vi "main.vi"() -> ()   [LabVIEW 2012]
uses:
  <vilib>/SAPHIR/ViBox - XControls/XTab/XTab.xctl
  <vilib>/GPower/VIRegister/Library/Typedefs/RegisterType.ctl
  <vilib>/GPower/VIRegister/Library/QManager/CreateRegister.vi
  <vilib>/GPower/VIRegister/Library/SubVIs/FindRegisterData.vi
  <vilib>/GPower/VIRegister/Library/SubVIs/WriteSub.vi
  <vilib>/GPower/VIRegister/Library/QManager/ReleaseRegister.vi
  <vilib>/GPower/Error/Library/IsError.vi
  <vilib>/GPower/VIRegister/Library/QManager/ReleaseAll.vi
  <vilib>/GPower/VIRegister/Library/QManager/QManagerAction.vi
  <vilib>/GPower/VIRegister/Library/QManager/GetRegisterData.vi
  <vilib>/GPower/Error/Library/SetError.vi
  <vilib>/GPower/Error/Library/FilterCodes.vi
  <vilib>/GPower/Error/Library/Filter/FilterMulti.vi
  <vilib>/GPower/Error/Library/ErrorType.vi
  <vilib>/GPower/Error/Library/SplitAppended.vi
  <vilib>/GPower/Error/Library/SubVIs/ExplanationToError.vi
  src/top/gloable.vi
  <vilib>/GPower/VIRegister/Library/QManager/GetQName.vi
  <vilib>/GPower/VIRegister/Library/QManager/StartQManager.vi
  <vilib>/Utility/config.llb/Read Key (String).vi
  <vilib>/Utility/config.llb/Read Key (U32).vi
  <vilib>/Utility/error.llb/Trim Whitespace.vi
  <vilib>/dlg_ctls.llb/Space Constant.vi
  <vilib>/Utility/error.llb/Error Code Database.vi
  <vilib>/GPower/Error/Library/SubVIs/SetStatus.vi
  <vilib>/GPower/Error/Library/AppendErrors.vi
  <vilib>/GPower/Error/Library/Append/AppendSingle.vi
  <vilib>/GPower/VIRegister/VIRegister.lvlib
  <vilib>/Utility/config.llb/NI_LVConfig.lvlib
panel:
  in  "XTab":refnum<vi>(xcontrol)
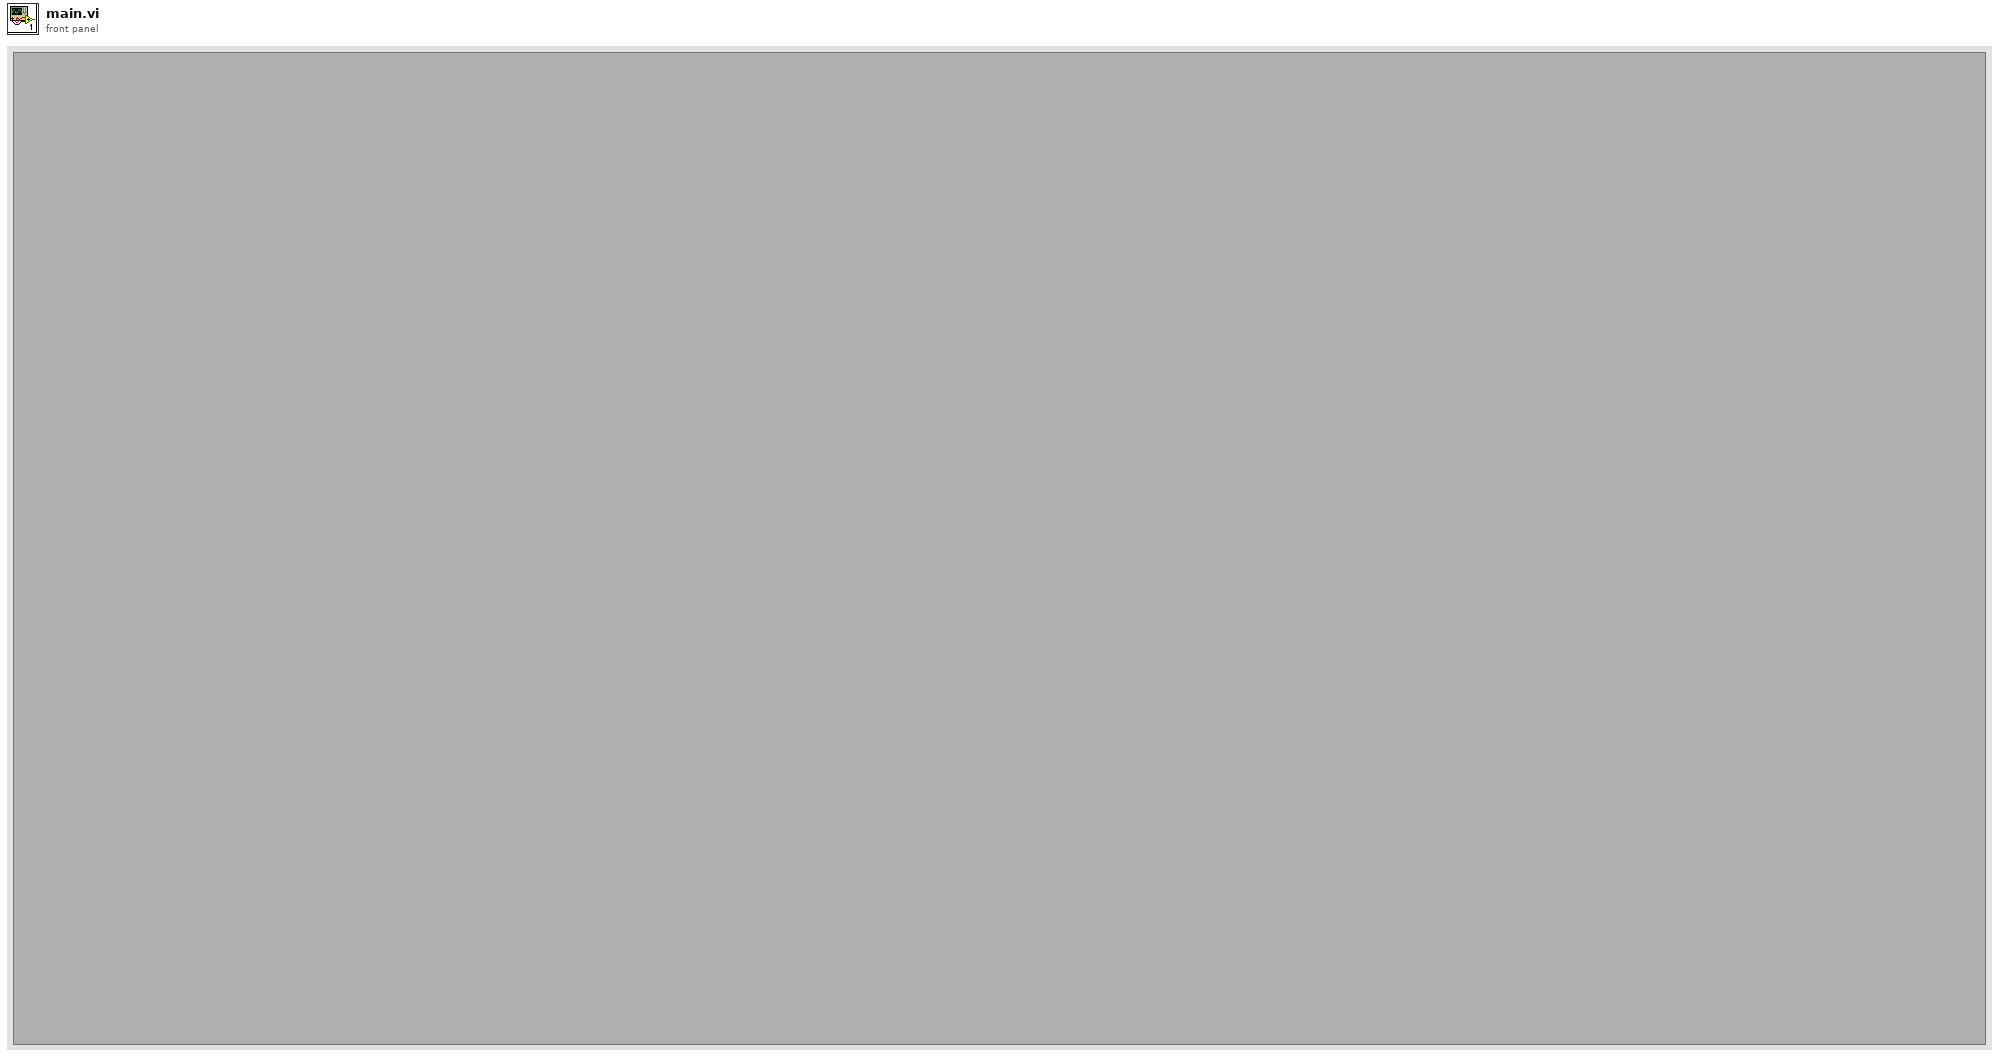
[diagram p1: front panel]
types:
  T1 = enum32{"invalid app kind", "Development System", "Run Time System", "Student Edition", "Embedded LabVIEW", "Evaluation", "Custom"}
  T2 = cluster{" 数据帧名称":string, " 数据":string, "备用操作符":bool, "起始地址":i32, "读写标志":i32, "长度":i32}
  T3 = enum32{"Invalid", "Standard", "Closed", "Hidden", "Minimized", "Maximized"}
  T4 = cluster{"Core":cluster{"Current VI Reference":refnum<vi>, "Close Panel on Exit?":bool}, "事件注册引用句柄":refnum<event-registration>, "XTab":refnum<vi>, "线程数组":refnum<vi>[], "通讯线程":refnum<vi>, "notifier out":refnum<notifier>, "sample_page":refnum<vi>, "queue out":refnum<queue>, "板卡":u32[], "txt引用":refnum<vi>}
  T5 = cluster{"Core":cluster{"Current VI Reference":refnum<vi>, "Close Panel on Exit?":bool}, "事件注册引用句柄":refnum<event-registration>, "XTab":refnum<vi>, "main_page":refnum<vi>, "earth_catch":refnum<vi>, "notifier out":refnum<notifier>, "sample_page":refnum<vi>}
  T6 = cluster{"Current VI Reference":refnum<vi>, "Close Panel on Exit?":bool}
  T7 = typedef "VIRegister.lvlib/RegisterType.ctl" = enum16{"Circular buffer", "FIFO buffer", "LIFO buffer", "Register"}
  T8 = typedef "NI_LVConfig.lvlib/Config Data RefNum.ctl" = refnum<k1>
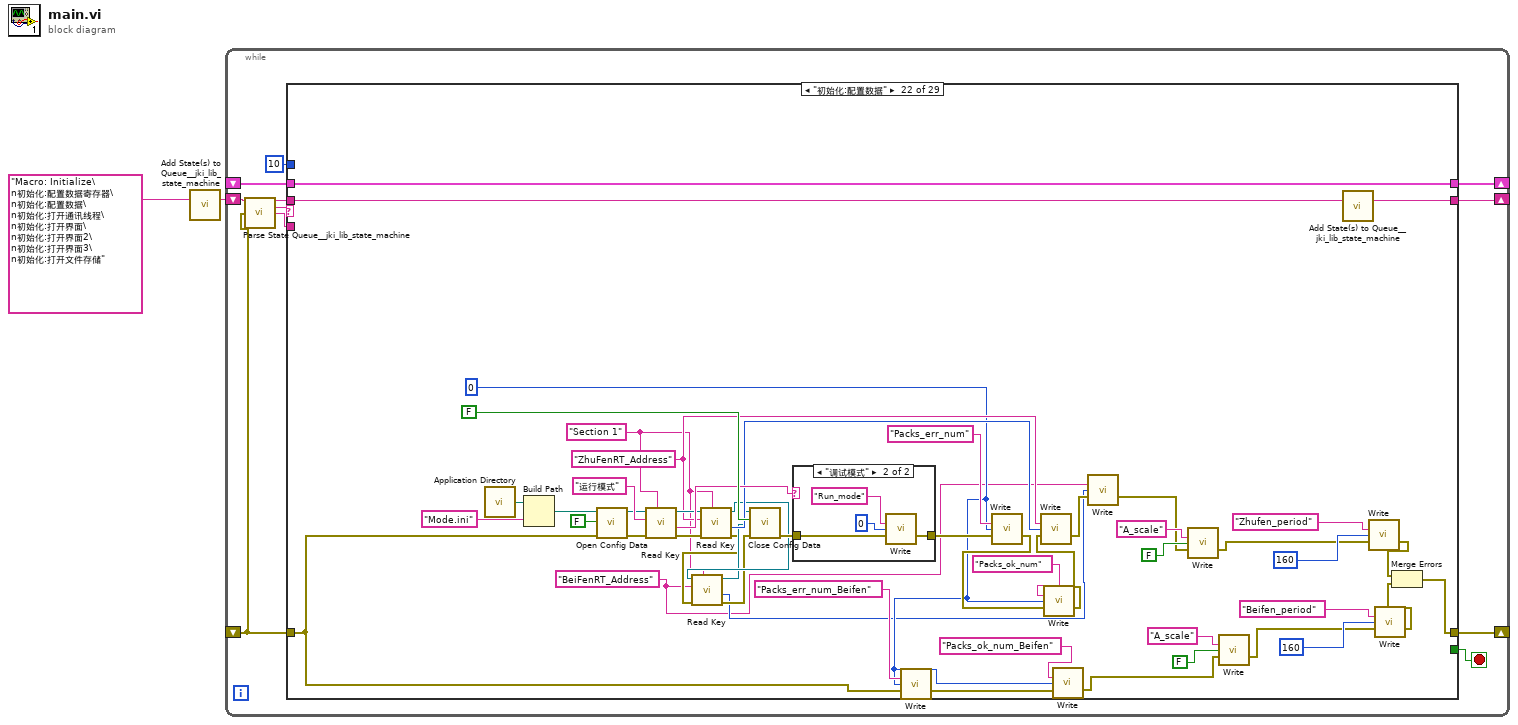
[diagram p0: block diagram]
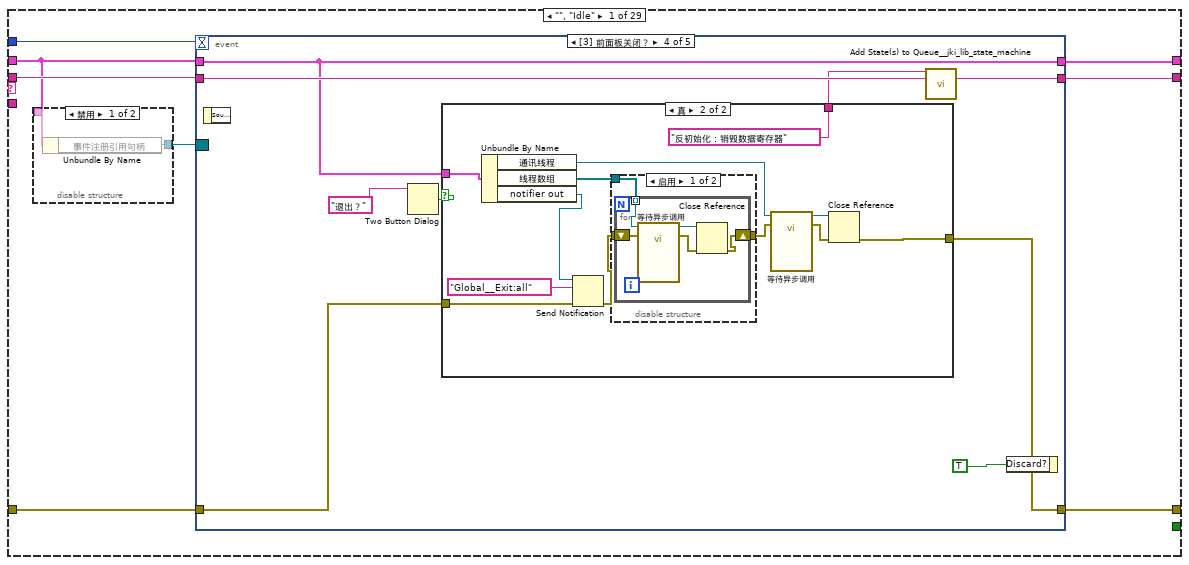
[diagram p2: hidden frame]
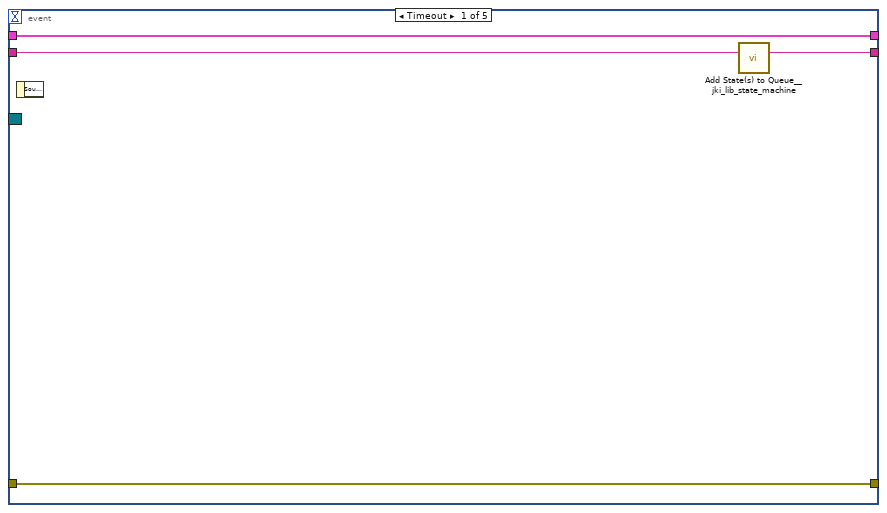
[diagram p4: hidden frame]
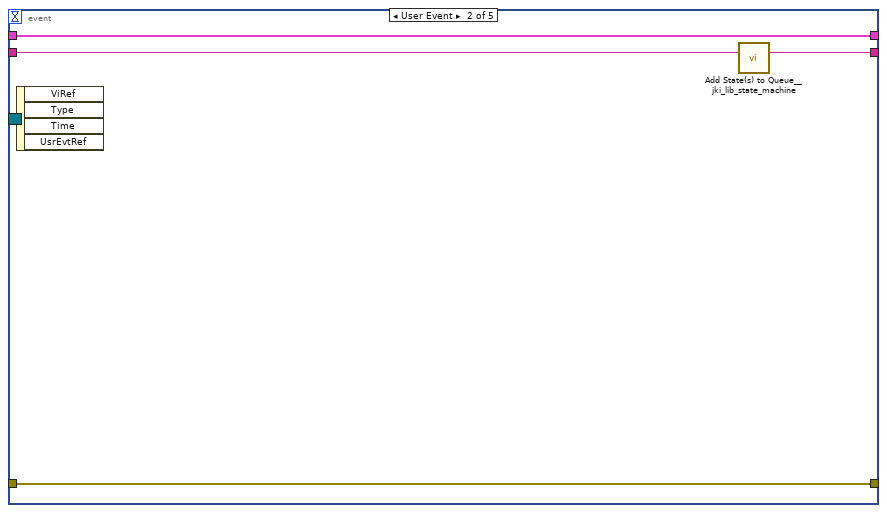
[diagram p5: hidden frame]
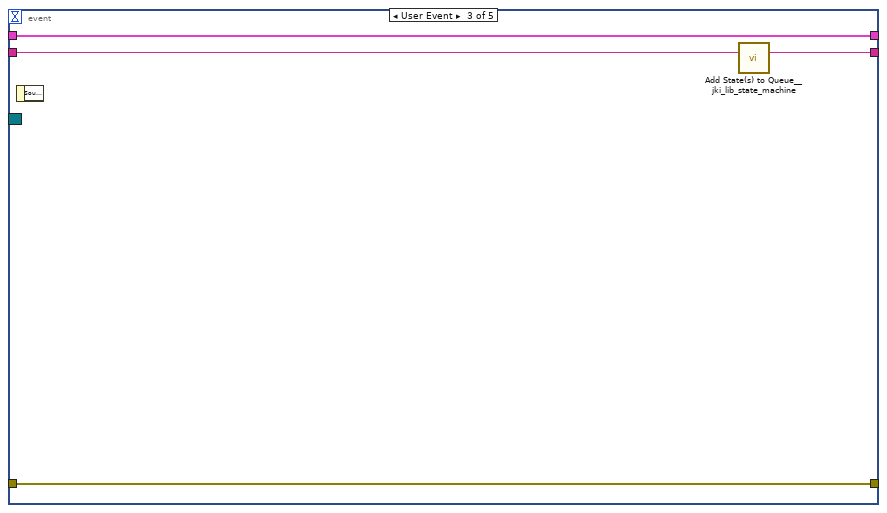
[diagram p6: hidden frame]
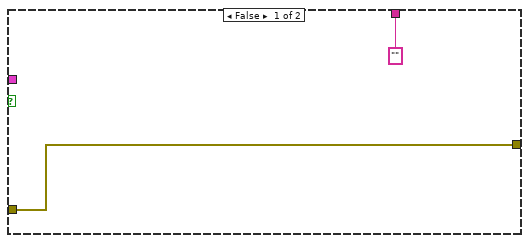
[diagram p7: hidden frame]
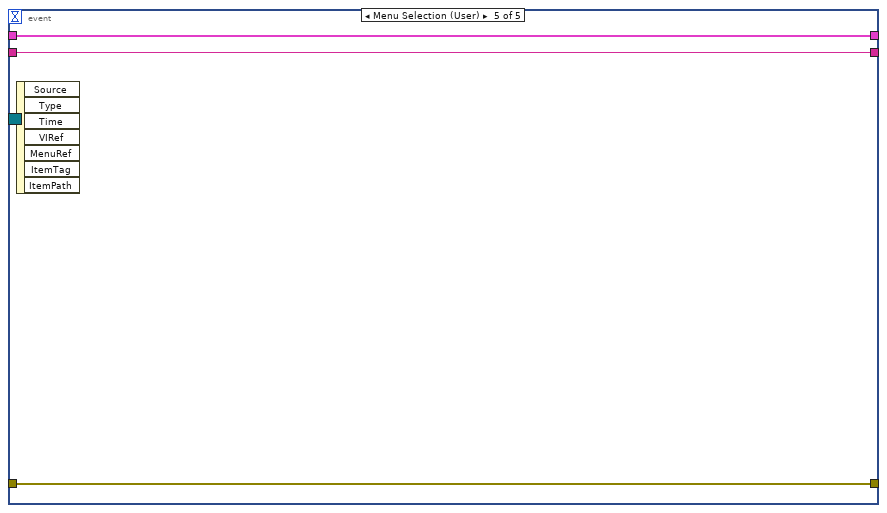
[diagram p9: hidden frame]
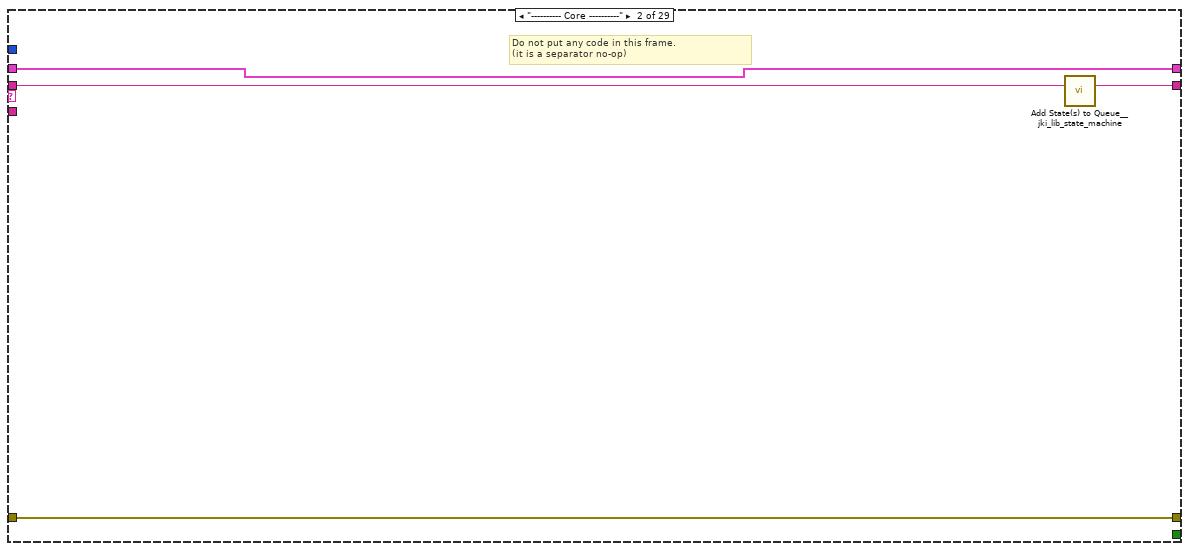
[diagram p10: hidden frame]
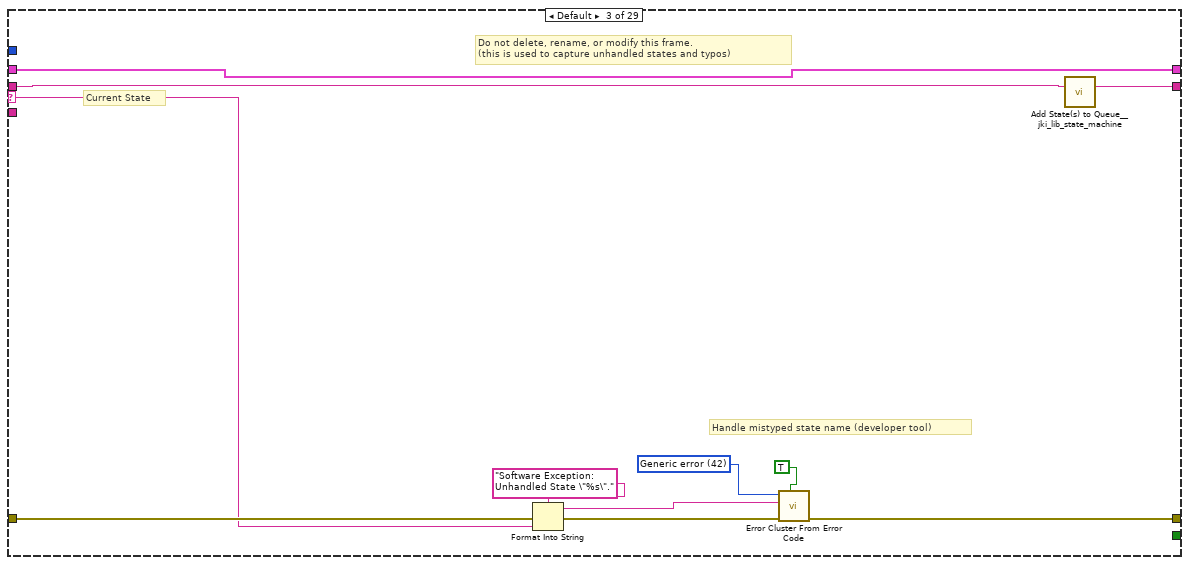
[diagram p11: hidden frame]
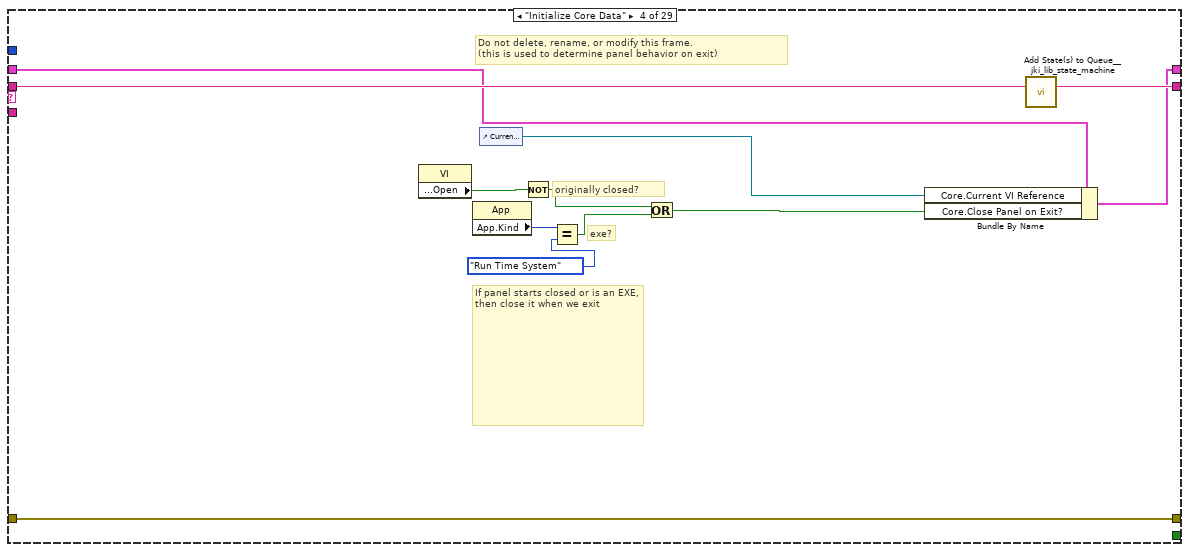
[diagram p12: hidden frame]
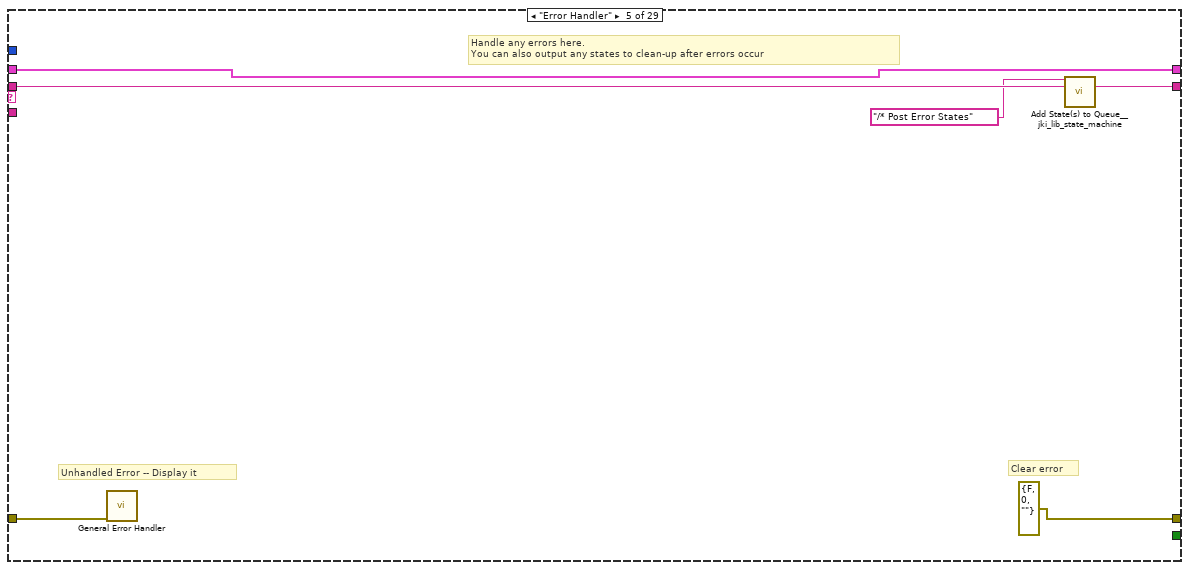
[diagram p13: hidden frame]
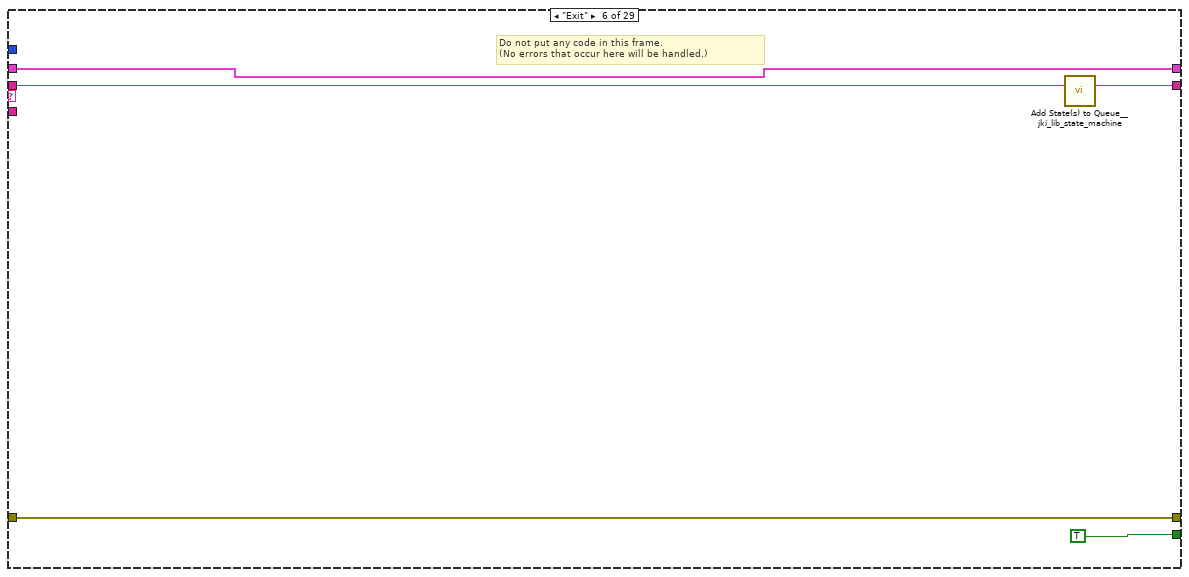
[diagram p14: hidden frame]
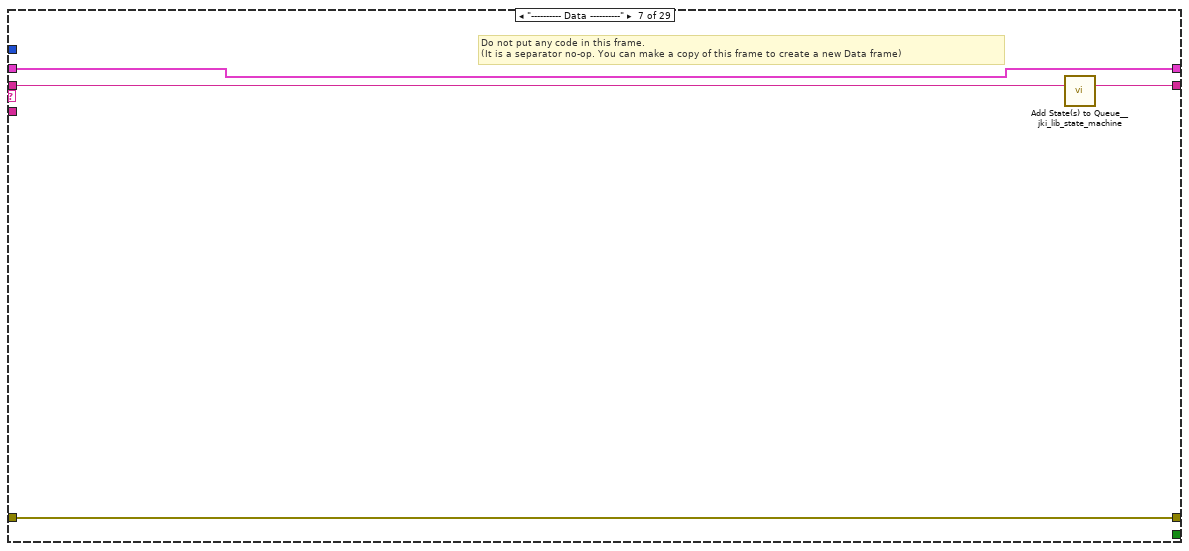
[diagram p15: hidden frame]
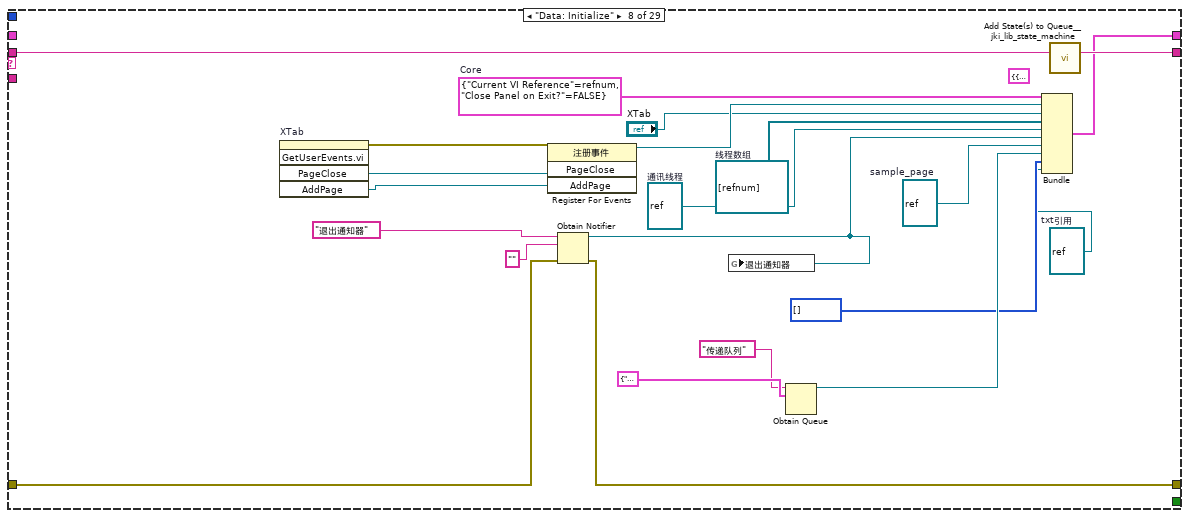
[diagram p16: hidden frame]
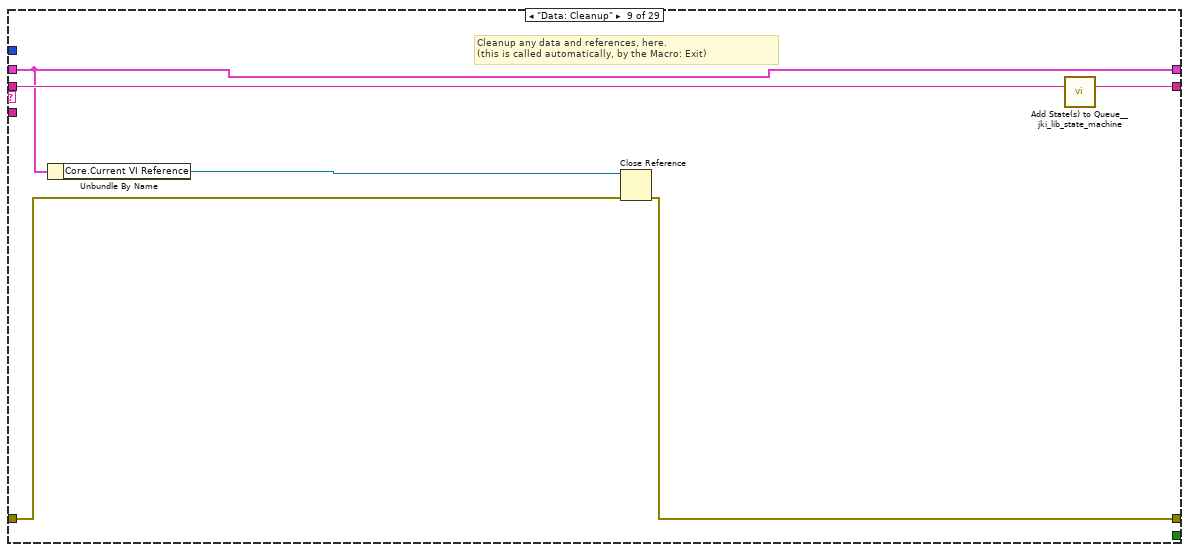
[diagram p17: hidden frame]
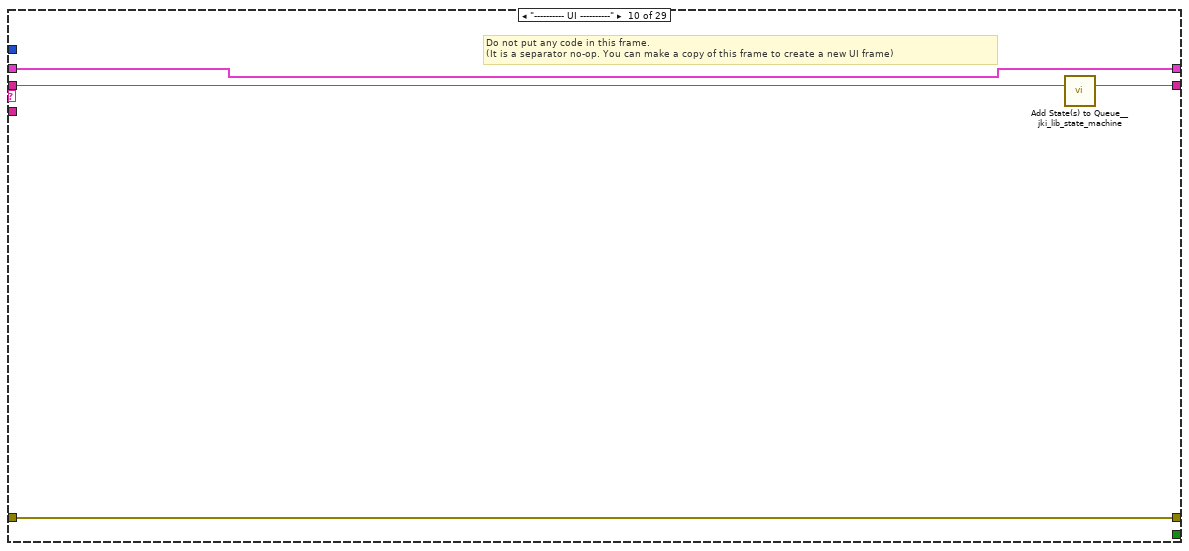
[diagram p18: hidden frame]
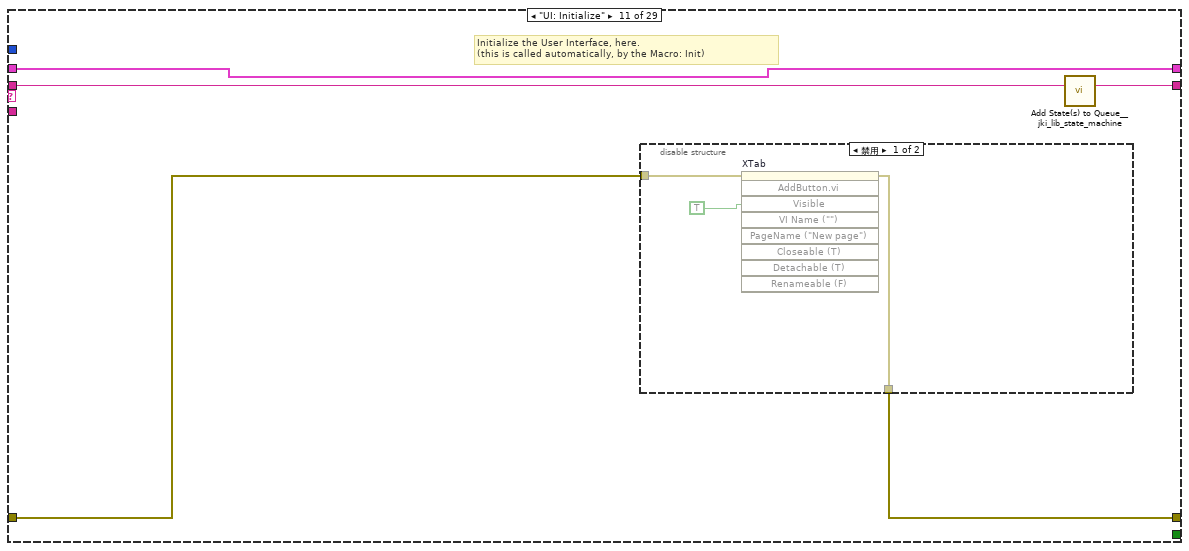
[diagram p19: hidden frame]
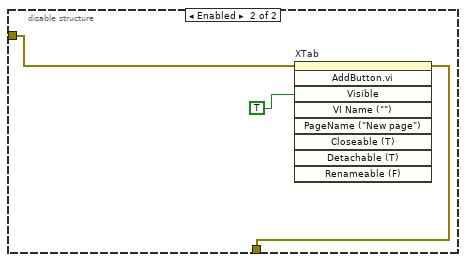
[diagram p20: hidden frame]
diagram:
  n1 = call <vilib>:"Add State(s) to Queue__jki_lib_state_machine.vi"("State(s) in (\"\")"="Macro: Initialize\n初始化:配置数据寄存器\n初始化:配置数据\n初始化:打开通讯线程\n初始化:打开界面\n初始化:打开界面2\n初始化:打开界面3\n初始化:打开文件存储") -> ("States Out"=w2:string)  [unwired: 14 in]
  n2 = while "JKI - String-Based Queued State Machine (Basic) v1.0" {
    shift-right: [w6] -> _
    shift-left: _ -> [w5]
    shift-right: [w9] -> _
    shift-left: _ -> [w3]
    shift-right: [w8] -> _
    shift-left: w2 -> [w10]
    stop <- w7 stop-if-true
    n3 = call <vilib>:"Parse State Queue__jki_lib_state_machine.vi"("State Queue"=w10, "Error In (no error)"=w3) -> ("Remaining States"=w12:string, "Current State"=w13:string, "Arguments"=w11:string)  [unwired: 11 in]
    n4 = case shown="\"初始化:配置数据\"" w13 {
      selector: w13 -> [_ _ w75 _ _ _ _ _ _ _ _ _ _ _ _ _ _ _ _ _ _ _ _ _ _ _ _ _ _]
      tunnel: w12 -> [w21 w74 w79 w97 w103 w108 w112 w134 w140 w144 w149 w161 w172 w196 w211 w225 w234 w239 w249 w253 w317 w367 w395 w421 w447 w470 w489 w495 w524]
      tunnel: w11 -> [_ _ _ _ _ _ _ _ _ _ _ w156 w166 _ _ _ _ _ _ _ _ _ _ _ _ _ _ _ _]
      tunnel: w5 -> [w15 w71 w77 w88 w100 w106 w109 _ w135 w141 w147 w159 w168 w197 w202 w222 w231 w236 w246 w250 w315 w365 w392 w418 w444 w468 w487 w492 w522]
      tunnel: [w19 w72 w81 w94 errorcluster {"status"=FALSE, "code"=0, "source"=""} ("error out") w105 w110 w123 w136 w142 w145 w157 w169 w195 w200 w221 w232 w237 w247 w251 w264 w327 w391 w417 w443 w465 w484 w493 w513] -> w9
      tunnel: w3 -> [w18 w72 w80 w94 w99 w105 w110 w122 w137 w142 w146 w158 w170 w195 w204 w224 w232 w237 w247 w251 w285 w335 w389 w415 w441 w464 w483 w493 w503]
      tunnel: [w20 w73 w78 w96 w102 w107 w111 w133 w139 w143 w148 w160 w171 w198 w212 w226 w233 w238 w248 w252 w316 w366 w394 w420 w446 w469 w488 w494 w523] -> w8
      tunnel: [_ _ _ _ _ TRUE _ _ _ _ _ _ _ _ _ _ _ _ _ _ _ _ _ _ _ _ _ _ _] -> w7
      tunnel: [w17 w71 w77 w95 w100 w106 w109 w132 w135 w141 w147 w159 w168 w197 w203 w222 w231 w236 w246 w250 w315 w365 w393 w419 w445 w466 w485 w492 w522] -> w6
      tunnel: 10 ("Timeout") -> [w16 _ _ _ _ _ _ _ _ _ _ _ _ _ _ _ _ _ _ _ _ _ _ _ _ _ _ _ _]
      frame "", "Idle" {
        n5 = disable-structure shown="禁用" {
          disable-tunnel: w15 -> [w23 _]
          disable-tunnel: [w22 _] -> w14
          frame Disabled {
            n6 = Unbundle By Name(w23) -> ("事件注册引用句柄"=w22:refnum<event-registration>)
          }
          frame Enabled {
          }
        }
        n7 = event shown="[3] 前面板关闭？" {
          selector: w14 -> [_ _ _ _ _]
          dyn-events: _ -> [_ _ _ _ _]
          timeout: w16 -> [_ _ _ _ _]
          tunnel: w21 -> [w27 w31 w35 w44 w69]
          tunnel: [w26 w30 w34 w43 w69] -> w20
          tunnel: w15 -> [w24 w28 w33 w40 w70]
          tunnel: [w25 w29 w32 w39 w68] -> w19
          tunnel: w18 -> [w25 w29 w32 w38 w68]
          tunnel: [w24 w28 w33 w40 w70] -> w17
          event Timeout {
            n8 = event-data() -> ()  [unwired: 1 in, 1 out]
            n9 = call <vilib>:"Add State(s) to Queue__jki_lib_state_machine.vi"("State(s) in (\"\")"=w27) -> ("States Out"=w26:string)  [unwired: 14 in]
          }
          event User Event {
            n10 = event-data() -> ()  [unwired: 1 in, 4 out]
            n11 = call <vilib>:"Add State(s) to Queue__jki_lib_state_machine.vi"("State(s) in (\"\")"=w31) -> ("States Out"=w30:string)  [unwired: 14 in]
          }
          event User Event {
            n12 = event-data() -> ()  [unwired: 1 in, 1 out]
            n13 = call <vilib>:"Add State(s) to Queue__jki_lib_state_machine.vi"("State(s) in (\"\")"=w35) -> ("States Out"=w34:string)  [unwired: 14 in]
          }
          event Panel Close? {
            n14 = event-data() -> ()  [unwired: 1 in, 1 out]
            n15 = Two Button Dialog(message="退出？" ("消息")) -> (T button?=w36:bool)  [unwired: 2 in]
            n16 = case shown="真" w36 {
              tunnel: ["" "反初始化：销毁数据寄存器"] -> w42
              tunnel: w40 -> [_ w57]
              tunnel: [w45 w49] -> w39
              tunnel: w38 -> [w45 w54]
              frame False {
              }
              frame True {
                n17 = Unbundle By Name(w57) -> ("通讯线程"=w51:refnum<vi>, "线程数组"=w47:refnum<vi>[], "notifier out"=w56:refnum<notifier>)
                n18 = Send Notification(notification="Global__Exit:all" ("通知"), notifier=w56, error in (no error)=w54) -> (error out=w48:errorcluster)  [unwired: 1 out]
                n19 = disable-structure shown="启用" {
                  disable-tunnel: [w61 w67] -> w50
                  disable-tunnel: w48 -> [w60 w67]
                  disable-tunnel: w47 -> [w59 _]
                  frame Enabled {
                    n20 = for {
                      shift-right: [w64] -> w61
                      shift-left: w60 -> [w63]
                      tunnel: w59 -> [w62] mode=indexing
                      n21 = call-by-ref "等待异步调用"(reference=w62, error in=w63) -> (reference out=w65:refnum<vi>, error out=w66:errorcluster)  [unwired: 12 in]
                      n22 = Close Reference(reference=w65, error in (no error)=w66) -> (error out=w64:errorcluster)
                    }
                  }
                  frame Disabled {
                  }
                }
                n23 = call-by-ref "等待异步调用"(reference=w51, error in=w50) -> (reference out=w53:refnum<vi>, error out=w52:errorcluster)  [unwired: 12 in]
                n24 = Close Reference(reference=w53, error in (no error)=w52) -> (error out=w49:errorcluster)
              }
            }
            n25 = call <vilib>:"Add State(s) to Queue__jki_lib_state_machine.vi"("State(s) in Front (\"\")"=w42, "State(s) in (\"\")"=w44) -> ("States Out"=w43:string)  [unwired: 13 in]
            n26 = event-data("Discard?"=TRUE) -> ()  [unwired: 1 in, 1 out]
          }
          event Menu Selection (User) {
            n27 = event-data() -> ()  [unwired: 1 in, 7 out]
          }
        }
      }
      frame "---------- Core ----------" {
        # "Do not put any code in this frame.\n(it is a separator no-op)"
        n28 = call <vilib>:"Add State(s) to Queue__jki_lib_state_machine.vi"("State(s) in (\"\")"=w74) -> ("States Out"=w73:string)  [unwired: 14 in]
      }
      frame Default {
        w84 = 42 items=["No error", "Argument error", "Memory is full", "Out of zone", "End of file", "File already open", "Generic file I/O error", "File not found", "File permission error", "Disk is full", "Duplicate path", "Too many files open", "System feature not enabled", "Resource file not found", "Cannot add resource", "Resource not found", "Image not found", "Image memory error", "Pen does not exist", "Config type invalid", "Config token not found", "Config parse error", "Config memory error", "Bad external code format", "Bad external code offset", "External code not present", "Null window", "Destroy window error", "Null menu", "Print aborted", "Bad print record", "Print driver error", "Windows error during printing", "Memory error during printing", "Print dialog error", "Generic print error", "Invalid device refnum", "Device not found", "Device parameter error", "Device unit error", "Cannot open device", "Device call aborted", "Generic error", "Cancelled by user", "Object ID too low", "Object ID too high", "Object not in heap", "Unknown heap", "Unknown object (invalid DefProc)", "Unknown object (DefProc not in table)", "Message out of range", "Invalid (null) method", "Unknown message", "Manager call not supported", "Bad address", "Network operation in progress", "Network operation timed out", "Connection is busy", "Network attribute not supported", "Network error", "Address in use", "System out of memory", "Connection aborted", "Connection refused", "Not connected", "Already connected", "Connection closed", "Initialization error (interapplication manager)", "Bad occurrence", "Wait on unbound occurrence handler", "Occurrence queue overflow", "Datalog type conflict", "Unused", "Unrecognized type (interapplication manager)", "Memory corrupt", "Failed to make temporary DLL", "Old CIN version", "Drag socket not found", "Failed to load drop-object", "Failed to register OLE object", "Failed to release OLE object", "Format specifier type mismatch", "Unknown format specifier", "Too few format specifiers", "Too many format specifiers", "Scan failed", "Newer CIN version", "Error converting to variant", "Runtime menu error", "Password tampered", "Variant attribute not found", "Incompatible variant data type", "Event data is not available", "Event Store is not present", "Occurrence is not found", "Event Queue is not created", "Event info is not available", "Refnum passed is NULL", "Error retrieving Class GUID", "Error retrieving CoClass GUID", "Error retrieving TypeLib GUID.", "Bad built application magic bytes.", "Specific driver is different from the specific driver associated with the Logical Name.", "There is no session opened to the class driver.", "Max Error", "MAX - Error with config objects", "MAX - Error loading configuration", "MAX - Group not supported"]
        # "Current State"
        # "Do not delete, rename, or modify this frame.\n(this is used to capture unhandled states and typos)"
        # "Handle mistyped state name (developer tool)"
        n29 = Format Into String(format string="Software Exception: Unhandled State \"%s\"." ("message"), error in=w80, w75) -> (resulting string=w83:string, error out=w82:errorcluster)  [unwired: 1 in]
        n30 = call <vilib>:"Error Cluster From Error Code.vi"("show call chain? (False)"=TRUE, "error in (no error)"=w82, "error message (\"\")"=w83, "error code (0)"=w84) -> ("error out"=w81:errorcluster)  [unwired: 5 in]
        n31 = call <vilib>:"Add State(s) to Queue__jki_lib_state_machine.vi"("State(s) in (\"\")"=w79) -> ("States Out"=w78:string)  [unwired: 14 in]
      }
      frame "Initialize Core Data" {
        # "Do not delete, rename, or modify this frame.\n(this is used to determine panel behavior on exit)"
        # "originally closed?"
        # "exe?"
        # "If panel starts closed or is an EXE, then close it when we exit"
        n32 = property class="VI"() -> ("Front Panel.Open"=w93:bool)  [unwired: 2 in, 2 out]
        n33 = property class="App"() -> ("App.Kind"=w92:T1)  [unwired: 2 in, 2 out]
        n34 = control-ref of="Current VI Reference"() -> (w86:refnum<vi>)
        n35 = Not(x=w93) -> (.not. x?=w90:bool)
        n36 = Equal?(x=w92, y=T1."Run Time System" ("Application:Kind")) -> (x = y?=w89:bool)
        n37 = Or(x=w90, y=w89) -> (x .or. y?=w87:bool)
        n38 = Bundle By Name(cluster=w88, "Core.Current VI Reference"=w86, "Core.Close Panel on Exit?"=w87) -> (w95:T4)
        n39 = call <vilib>:"Add State(s) to Queue__jki_lib_state_machine.vi"("State(s) in (\"\")"=w97) -> ("States Out"=w96:string)  [unwired: 14 in]
      }
      frame "Error Handler" {
        # "Unhandled Error -- Display it"
        # "Handle any errors here.\nYou can also output any states to clean-up after errors occur"
        # "Clear error"
        n40 = call <vilib>:"General Error Handler.vi"("error in (no error)"=w99) -> ()  [unwired: 10 in, 5 out]
        n41 = call <vilib>:"Add State(s) to Queue__jki_lib_state_machine.vi"("State(s) in Front (\"\")"="/* Post Error States", "State(s) in (\"\")"=w103) -> ("States Out"=w102:string)  [unwired: 13 in]
      }
      frame "Exit" {
        # "Do not put any code in this frame.\n(No errors that occur here will be handled.)"
        n42 = call <vilib>:"Add State(s) to Queue__jki_lib_state_machine.vi"("State(s) in (\"\")"=w108) -> ("States Out"=w107:string)  [unwired: 14 in]
      }
      frame "---------- Data ----------" {
        # "Do not put any code in this frame.\n(It is a separator no-op. You can make a copy of this frame to create a new Data frame)"
        n43 = call <vilib>:"Add State(s) to Queue__jki_lib_state_machine.vi"("State(s) in (\"\")"=w112) -> ("States Out"=w111:string)  [unwired: 14 in]
      }
      frame "Data: Initialize" {
        w113 = refnum<vi> refnum  # txt引用
        w114 = refnum<vi>[] [refnum]  # 线程数组
        w116 = refnum<vi> refnum  # 通讯线程
        (unwired) T5 {"Core"={"Current VI Reference"=refnum, "Close Panel on Exit?"=FALSE}, "事件注册引用句柄"=refnum, "XTab"=refnum, "main_page"=refnum, "earth_catch"=refnum, "notifier out"=refnum, "sample_page"=refnum} ("输出簇")
        w121 = refnum<vi> refnum  # sample_page
        w131 = T6 {"Current VI Reference"=refnum, "Close Panel on Exit?"=FALSE}  # Core
        n44 = invoke on="XTab" class="XTab (strict)" method="GetUserEvents.vi"() -> (error out=w129:errorcluster, "PageClose"=w130:refnum<user-event>, "AddPage"=w128:refnum<user-event>)  [unwired: 5 in, 2 out]
        n45 = register-events(error in=w129, w130, w128) -> (reference out=w127:refnum<event-registration>)  [unwired: 1 in, 1 out]
        n46 = Obtain Notifier(name (unnamed)="退出通知器" ("名称（未命名）"), notification data type="" ("名称（未命名）"), error in (no error)=w122) -> (notifier out=w120:refnum<notifier>, error out=w123:errorcluster)  [unwired: 1 in, 1 out]
        n47 = global write "gloable.vi" "退出通知器"(w120) -> ()
        n48 = Obtain Queue(name (unnamed)="传递队列" ("名称（未命名）"), element data type=T2 {" 数据帧名称"="", " 数据"="", "备用操作符"=TRUE, "起始地址"=0, "读写标志"=0, "长度"=0}) -> (queue out=w117:refnum<queue>)  [unwired: 3 in, 2 out]
        n49 = Bundle("Core"=w131, "事件注册引用句柄"=w127, "XTab"="XTab", "线程数组"=w114, "通讯线程"=w116, "notifier out"=w120, "sample_page"=w121, "queue out"=w117, "板卡"=u32[] [], "txt引用"=w113) -> (w132:T4)  [unwired: 1 in]
        n50 = call <vilib>:"Add State(s) to Queue__jki_lib_state_machine.vi"("State(s) in (\"\")"=w134) -> ("States Out"=w133:string)  [unwired: 14 in]
      }
      frame "Data: Cleanup" {
        # "Cleanup any data and references, here.\n(this is called automatically, by the Macro: Exit)"
        n51 = Unbundle By Name(w135) -> ("Core.Current VI Reference"=w138:refnum<vi>)
        n52 = Close Reference(reference=w138, error in (no error)=w137) -> (error out=w136:errorcluster)
        n53 = call <vilib>:"Add State(s) to Queue__jki_lib_state_machine.vi"("State(s) in (\"\")"=w140) -> ("States Out"=w139:string)  [unwired: 14 in]
      }
      frame "---------- UI ----------" {
        # "Do not put any code in this frame.\n(It is a separator no-op. You can make a copy of this frame to create a new UI frame)"
        n54 = call <vilib>:"Add State(s) to Queue__jki_lib_state_machine.vi"("State(s) in (\"\")"=w144) -> ("States Out"=w143:string)  [unwired: 14 in]
      }
      frame "UI: Initialize" {
        # "Initialize the User Interface, here.\n(this is called automatically, by the Macro: Init)"
        n55 = disable-structure shown="禁用" {
          disable-tunnel: w146 -> [w151 w153]
          disable-tunnel: [w150 w155] -> w145
          frame Disabled {
            n56 = invoke on="XTab" class="XTab (strict)" method="AddButton.vi"(error in=w151, "Visible"=TRUE) -> (error out=w150:errorcluster)  [unwired: 7 in, 8 out]
          }
          frame Enabled {
            n57 = invoke on="XTab" class="XTab (strict)" method="AddButton.vi"(error in=w153, "Visible"=TRUE) -> (error out=w155:errorcluster)  [unwired: 7 in, 8 out]
          }
        }
        n58 = call <vilib>:"Add State(s) to Queue__jki_lib_state_machine.vi"("State(s) in (\"\")"=w149) -> ("States Out"=w148:string)  [unwired: 14 in]
      }
      frame "UI: Cursor Set" {
        # "Argument"
        # "Set and Unset Cursor Busy.\n(Usage: \"UI: Cursor Set >> Busy|Idle\")"
        n59 = case shown="\"Busy\"" w156 {
          tunnel: w158 -> [w163 w165]
          tunnel: [w162 w164] -> w157
          frame "Idle", Default {
            n60 = call <vilib>:"Unset Busy.vi"("error in (no error)"=w163) -> ("error out"=w162:errorcluster)  [unwired: 10 in]
          }
          frame "Busy" {
            n61 = call <vilib>:"Set Busy.vi"("error in (no error)"=w165) -> ("error out"=w164:errorcluster)  [unwired: 9 in, 1 out]
          }
        }
        n62 = call <vilib>:"Add State(s) to Queue__jki_lib_state_machine.vi"("State(s) in (\"\")"=w161) -> ("States Out"=w160:string)  [unwired: 14 in]
      }
      frame "UI: Front Panel State" {
        # "Argument"
        # "Set Front Panel Open or Closed\n(Usage: \"UI: Front Panel State >> Open|Close\")"
        n63 = Unbundle By Name(w168) -> ("Core.Current VI Reference"=w167:refnum<vi>)
        n64 = case shown="\"Open\", 默认" w166 {
          tunnel: w170 -> [w176 w189]
          tunnel: [w178 w190] -> w169
          tunnel: w167 -> [w177 w187]
          frame "Open", Default {
            n65 = property class="VI"(reference=w177, error in=w176) -> (reference out=w174:refnum<vi>, error out=w175:errorcluster, "Front Panel.Open"=w173:bool)
            n66 = case shown="假" w173 {
              tunnel: [w181 w184] -> w178
              tunnel: w175 -> [w180 w184]
              tunnel: w174 -> [w179 _]
              frame False {
                n67 = invoke class="VI" method="FP.Open"(reference=w179, error in=w180, "Activate"=FALSE, "State"=T3."Hidden") -> (error out=w181:errorcluster)  [unwired: 1 in, 4 out]
              }
              frame True {
              }
            }
          }
          frame "Close" {
            n68 = property class="VI"(reference=w187, error in=w189) -> (reference out=w186:refnum<vi>, error out=w188:errorcluster, "Front Panel.Open"=w185:bool)
            n69 = case shown="真" w185 {
              tunnel: [w191 w194] -> w190
              tunnel: w188 -> [w191 w193]
              tunnel: w186 -> [_ w192]
              frame False {
              }
              frame True {
                n70 = invoke class="VI" method="FP.Close"(reference=w192, error in=w193) -> (error out=w194:errorcluster)  [unwired: 1 in, 2 out]
              }
            }
          }
        }
        n71 = call <vilib>:"Add State(s) to Queue__jki_lib_state_machine.vi"("State(s) in (\"\")"=w172) -> ("States Out"=w171:string)  [unwired: 14 in]
      }
      frame "---------- Hardware ----------" {
        # "Do not put any code in this frame.\n(It is a separator no-op. You can make a copy of this frame to create a new UI frame)"
        n72 = call <vilib>:"Add State(s) to Queue__jki_lib_state_machine.vi"("State(s) in (\"\")"=w196) -> ("States Out"=w198:string)  [unwired: 14 in]
      }
      frame "Hardware: Initialize" {
        n73 = call "bs Base Init Cards.vi"("error in (no error)"=w204) -> ("error out"=w210:errorcluster)  [unwired: 10 in]
        n74 = call "bs Base Find Cards For LabView.vi"("error in (no error)"=w210, "IP"="") -> ("error out"=w206:errorcluster, "RsrcInf[]"=w209:string[][])  [unwired: 8 in]
        n75 = Index Array(array=w209, index (col)=5 ("禁用的索引 (列)")) -> (element=w207:string[])  [unwired: 1 in]
        n76 = for {
          tunnel: w207 -> [w220] mode=indexing
          shift-right: [w218] -> w199
          shift-left: w206 -> [w219]
          tunnel: [w217] -> w201 mode=indexing
          n77 = call "bs Base Open Card.vi"("error in (no error)"=w219, "pInstrDesc"=w220) -> ("error out"=w218:errorcluster, "pInstr"=w217:u32)  [unwired: 8 in]
        }
        n78 = for {
          tunnel: w201 -> [w214] mode=indexing
          tunnel: [w215] -> w200
          tunnel: w199 -> [w213]
          n79 = call "bs Base Set IP.vi"("error in (no error)"=w213, "EnIsoPower"=TRUE, "instr"=w214) -> ("error out"=w215:errorcluster)  [unwired: 7 in, 1 out]
        }
        n80 = Bundle By Name(cluster=w202, "板卡"=w201) -> (w203:T4)
        n81 = call <vilib>:"Add State(s) to Queue__jki_lib_state_machine.vi"("State(s) in (\"\")"=w211) -> ("States Out"=w212:string)  [unwired: 14 in]
      }
      frame "Hardware: Cleanup" {
        n82 = Unbundle By Name(w222) -> ("板卡"=w223:u32[])
        n83 = for {
          tunnel: w224 -> [w229]
          tunnel: w223 -> [w227] mode=indexing
          tunnel: [w228] -> w221
          n84 = call "bs Base Set IP.vi"("error in (no error)"=w229, "EnIsoPower"=FALSE, "instr"=w227) -> ("error out"=w228:errorcluster)  [unwired: 7 in, 1 out]
        }
        n85 = call <vilib>:"Add State(s) to Queue__jki_lib_state_machine.vi"("State(s) in (\"\")"=w225) -> ("States Out"=w226:string)  [unwired: 14 in]
      }
      frame "---------- Macro ----------" {
        # "Do not put any code in this frame.\n(It is a separator no-op. You can make a copy of this frame to create a new Macro frame)"
        n86 = call <vilib>:"Add State(s) to Queue__jki_lib_state_machine.vi"("State(s) in (\"\")"=w234) -> ("States Out"=w233:string)  [unwired: 14 in]
      }
      frame "Macro: Initialize" {
        # "Initialization Macro\n(This is called once, when the VI starts)"
        n87 = call <vilib>:"Add State(s) to Queue__jki_lib_state_machine.vi"("State(s) in Front (\"\")"="Data: Initialize\nInitialize Core Data\nUI: Initialize\nHardware: Initialize\nUI: Front Panel State >> Open", "State(s) in (\"\")"=w239) -> ("States Out"=w238:string)  [unwired: 13 in]
      }
      frame "Macro: Exit" {
        # "Exit Macro\n(This is called once, when the VI exits)"
        n88 = Unbundle By Name(w246) -> ("Core.Close Panel on Exit?"=w245:bool)
        n89 = Select(t="UI: Front Panel State >> Close", s=w245, f="") -> (s? t:f=w242:string)
        n90 = call <vilib>:"Add State(s) to Queue__jki_lib_state_machine.vi"("State(s) in (\"\")"=w242, "State(s) at Back (\"\")"="Data: Cleanup\nHardware: Cleanup\nExit") -> ("States Out"=w240:string)  [unwired: 13 in]
        n91 = call <vilib>:"Add State(s) to Queue__jki_lib_state_machine.vi"("State(s) in Front (\"\")"=w240, "State(s) in (\"\")"=w249) -> ("States Out"=w248:string)  [unwired: 13 in]
      }
      frame "---------- 初始化----------" {
        n92 = call <vilib>:"Add State(s) to Queue__jki_lib_state_machine.vi"("State(s) in (\"\")"=w253) -> ("States Out"=w252:string)  [unwired: 14 in]
      }
      frame "初始化:配置数据寄存器" {
        w258 = RegisterType."FIFO buffer" ("Register type")
        w254 = RegisterType."Register" ("Register type")
        # "只有全局数据在这里初始化寄存器"
        n93 = call <vilib>:"Create.vi"("Register name"="1553BBeiFenRecv", "Register type"=w258, "Error in"=w285) -> ("Error out"=w309:errorcluster)  [unwired: 11 in, 1 out]
        n94 = call <vilib>:"Create.vi"("Register name"="Packs_err_num", "Register type"=w254, "Error in"=w285) -> ("Error out"=w280:errorcluster)  [unwired: 11 in, 1 out]
        n95 = call <vilib>:"Create.vi"("Register name"="1553BZhuFenRecv", "Register type"=w258, "Error in"=w309) -> ("Error out"=w284:errorcluster)  [unwired: 11 in, 1 out]
        n96 = call <vilib>:"Create.vi"("Register name"="Packs_err_num_Beifen", "Register type"=w254, "Error in"=w280) -> ("Error out"=w279:errorcluster)  [unwired: 11 in, 1 out]
        n97 = call <vilib>:"Create.vi"("Register name"="FileCancel", "Register type"=w258, "Error in"=w284) -> ("Error out"=w283:errorcluster)  [unwired: 11 in, 1 out]
        n98 = call <vilib>:"Create.vi"("Register name"="FileCancel_Beifen", "Register type"=w258, "Error in"=w283) -> ("Error out"=w262:errorcluster)  [unwired: 11 in, 1 out]
        n99 = call <vilib>:"Create.vi"("Register name"="ZhuFenJiaDuanDianWord", "Register type"=w258, "Error in"=w262) -> ("Error out"=w260:errorcluster)  [unwired: 11 in, 1 out]
        n100 = call <vilib>:"Create.vi"("Register name"="BeiFenJiaDuanDianWord", "Register type"=w258, "Error in"=w260) -> ()  [unwired: 11 in, 2 out]
        n101 = call <vilib>:"Create.vi"("Register name"="DiJian_mode_Beifen", "Register type"=w254, "Error in"=w279) -> ("Error out"=w276:errorcluster)  [unwired: 11 in, 1 out]
        n102 = call <vilib>:"Create.vi"("Register name"="DiJian_data_Beifen", "Register type"=w254, "Error in"=w276) -> ("Error out"=w275:errorcluster)  [unwired: 11 in, 1 out]
        n103 = call <vilib>:"Create.vi"("Register name"="Beifen_on", "Register type"=w254, "Error in"=w275) -> ("Error out"=w263:errorcluster)  [unwired: 11 in, 1 out]
        n104 = call <vilib>:"Create.vi"("Register name"="AIs", "Register type"=w254, "Error in"=w263) -> ("Error out"=w312:errorcluster)  [unwired: 11 in, 1 out]
        n105 = call <vilib>:"Create.vi"("Register name"="DiJian_mode", "Register type"=w254, "Error in"=w312) -> ("Error out"=w311:errorcluster)  [unwired: 11 in, 1 out]
        n106 = call <vilib>:"Create.vi"("Register name"="DiJian_data", "Register type"=w254, "Error in"=w311) -> ("Error out"=w305:errorcluster)  [unwired: 11 in, 1 out]
        n107 = call <vilib>:"Create.vi"("Register name"="Zhufen_on", "Register type"=w254, "Error in"=w305) -> ("Error out"=w302:errorcluster)  [unwired: 11 in, 1 out]
        n108 = call <vilib>:"Create.vi"("Register name"="1553BBeiFenRecv_stat", "Register type"=w254, "Error in"=w302) -> ("Error out"=w301:errorcluster)  [unwired: 11 in, 1 out]
        n109 = call <vilib>:"Create.vi"("Register name"="Run_mode", "Register type"=w254, "Error in"=w301) -> ("Error out"=w300:errorcluster)  [unwired: 11 in, 1 out]
        n110 = call <vilib>:"Create.vi"("Register name"="1553BZhuFenRecv_stat", "Register type"=w254, "Error in"=w300) -> ("Error out"=w298:errorcluster)  [unwired: 11 in, 1 out]
        n111 = call <vilib>:"Create.vi"("Register name"="ZhuFenRT_Address", "Register type"=w254, "Error in"=w298) -> ("Error out"=w257:errorcluster)  [unwired: 11 in, 1 out]
        n112 = call <vilib>:"Create.vi"("Register name"="BeiFenRT_Address", "Register type"=w254, "Error in"=w257) -> ("Error out"=w256:errorcluster)  [unwired: 11 in, 1 out]
        n113 = call <vilib>:"Create.vi"("Register name"="A_scale", "Register type"=w254, "Error in"=w256) -> ("Error out"=w292:errorcluster)  [unwired: 11 in, 1 out]
        n114 = call <vilib>:"Create.vi"("Register name"="A_scale_Beifen", "Register type"=w254) -> ("Error out"=w268:errorcluster)  [unwired: 12 in, 1 out]
        n115 = call <vilib>:"Create.vi"("Register name"="A_sam_num", "Register type"=w254, "Error in"=w292) -> ("Error out"=w291:errorcluster)  [unwired: 11 in, 1 out]
        n116 = call <vilib>:"Create.vi"("Register name"="A_sam_num_Beifen", "Register type"=w254, "Error in"=w268) -> ("Error out"=w269:errorcluster)  [unwired: 11 in, 1 out]
        n117 = call <vilib>:"Create.vi"("Register name"="G_sam_num", "Register type"=w254, "Error in"=w291) -> ("Error out"=w289:errorcluster)  [unwired: 11 in, 1 out]
        n118 = call <vilib>:"Create.vi"("Register name"="G_sam_num_Beifen", "Register type"=w254, "Error in"=w269) -> ("Error out"=w271:errorcluster)  [unwired: 11 in, 1 out]
        n119 = call <vilib>:"Create.vi"("Register name"="Zhufen_period", "Register type"=w254, "Error in"=w289) -> ("Error out"=w286:errorcluster)  [unwired: 11 in, 1 out]
        n120 = call <vilib>:"Create.vi"("Register name"="Beifen_period", "Register type"=w254, "Error in"=w271) -> ("Error out"=w273:errorcluster)  [unwired: 11 in, 1 out]
        n121 = call <vilib>:"Create.vi"("Register name"="Packs_ok_num", "Register type"=w254, "Error in"=w286) -> ()  [unwired: 11 in, 2 out]
        n122 = call <vilib>:"Create.vi"("Register name"="Packs_ok_num_Beifen", "Register type"=w254, "Error in"=w273) -> ("Error out"=w264:errorcluster)  [unwired: 11 in, 1 out]
        n123 = call <vilib>:"Add State(s) to Queue__jki_lib_state_machine.vi"("State(s) in (\"\")"=w317) -> ("States Out"=w316:string)  [unwired: 14 in]
      }
      frame "初始化:配置数据" {
        w318 = "BeiFenRT_Address" ("Register name")
        w351 = "ZhuFenRT_Address" ("Register name")
        w331 = u32 0
        w322 = "Section 1" ("section")
        n124 = call <vilib>:"Application Directory.vi"() -> ("Application Directory"=w359:path)
        n125 = Build Path(base path=w359, name or relative path="Mode.ini" ("名称或相对路径")) -> (appended path=w357:path)
        n126 = call <vilib>:"Open Config Data.vi"("error in (no error)"=w335, "create file if necessary (T)"=FALSE ("create file if necessary? (T)"), "configuration file path"=w357) -> ("error out"=w363:errorcluster, "refnum"=w362:T8)  [unwired: 6 in, 1 out]
        n127 = call-poly <vilib>:"Read Key.vi"("section"=w322, "error in (no error)"=w363, "key"="运行模式" ("Key 1"), "refnum"=w362) -> ("error out"=w349:errorcluster, "value"=w356:string, "refnum out"=w352:T8)  [unwired: 2 in, 3 out]
        n128 = call-poly <vilib>:"Read Key.vi"("section"=w322, "error in (no error)"=w349, "key"=w351, "refnum"=w352) -> ("error out"=w324:errorcluster, "value"=w350:u32, "refnum out"=w326:T8)  [unwired: 1 in, 4 out]
        n129 = call-poly <vilib>:"Read Key.vi"("section"=w322, "error in (no error)"=w324, "key"=w318, "refnum"=w326) -> ("error out"=w323:errorcluster, "value"=w319:u32, "refnum out"=w325:T8)  [unwired: 1 in, 4 out]
        n130 = call <vilib>:"Close Config Data.vi"("error in (no error)"=w323, "write file if changed (T)"=FALSE ("write configuration file? (T)"), "refnum"=w325) -> ("error out"=w355:errorcluster)  [unwired: 8 out]
        n131 = case shown="\"调试模式\"" w356 {
          tunnel: w355 -> [w369 w372]
          tunnel: [w368 w373] -> w353
          frame "测试模式", Default {
            n132 = call <vilib>:"Write.vi"("Register name"="Run_mode", "Register value"=u8 1, "Error in"=w369) -> ("Error out"=w368:errorcluster)  [unwired: 10 in, 2 out]
          }
          frame "调试模式" {
            n133 = call <vilib>:"Write.vi"("Register name"="Run_mode", "Register value"=u8 0, "Error in"=w372) -> ("Error out"=w373:errorcluster)  [unwired: 10 in, 2 out]
          }
        }
        n134 = call <vilib>:"Write.vi"("Register name"="Packs_err_num_Beifen", "Register value"=w331, "Error in"=w335) -> ("Error out"=w334:errorcluster)  [unwired: 10 in, 2 out]
        n135 = call <vilib>:"Write.vi"("Register name"="Packs_err_num", "Register value"=w331, "Error in"=w353) -> ("Error out"=w342:errorcluster)  [unwired: 10 in, 2 out]
        n136 = call <vilib>:"Write.vi"("Register name"="Packs_ok_num", "Register value"=w331, "Error in"=w342) -> ("Error out"=w341:errorcluster)  [unwired: 10 in, 2 out]
        n137 = call <vilib>:"Write.vi"("Register name"=w351, "Register value"=w350, "Error in"=w341) -> ("Error out"=w321:errorcluster)  [unwired: 10 in, 2 out]
        n138 = call <vilib>:"Write.vi"("Register name"="Packs_ok_num_Beifen", "Register value"=w331, "Error in"=w334) -> ("Error out"=w333:errorcluster)  [unwired: 10 in, 2 out]
        n139 = call <vilib>:"Write.vi"("Register name"=w318, "Register value"=w319, "Error in"=w321) -> ("Error out"=w320:errorcluster)  [unwired: 10 in, 2 out]
        n140 = call <vilib>:"Write.vi"("Register name"="A_scale", "Register value"=FALSE, "Error in"=w320) -> ("Error out"=w344:errorcluster)  [unwired: 10 in, 2 out]
        n141 = call <vilib>:"Write.vi"("Register name"="A_scale", "Register value"=FALSE, "Error in"=w333) -> ("Error out"=w330:errorcluster)  [unwired: 10 in, 2 out]
        n142 = call <vilib>:"Add State(s) to Queue__jki_lib_state_machine.vi"("State(s) in (\"\")"=w367) -> ("States Out"=w366:string)  [unwired: 14 in]
        n143 = call <vilib>:"Write.vi"("Register name"="Zhufen_period", "Register value"=u16 160, "Error in"=w344) -> ("Error out"=w328:errorcluster)  [unwired: 10 in, 2 out]
        n144 = call <vilib>:"Write.vi"("Register name"="Beifen_period", "Register value"=u16 160, "Error in"=w330) -> ("Error out"=w329:errorcluster)  [unwired: 10 in, 2 out]
        n145 = Merge Errors(w328, w329) -> (w327:errorcluster)
      }
      frame "初始化:打开界面" {
        w376 = FALSE ("Closeable (T)")
        # "Your code here.\n(You can make a copy of, or modify, this frame)"
        n146 = Unbundle By Name(w392) -> ("线程数组"=w380:refnum<vi>[], "notifier out"=w390:refnum<notifier>, "queue out"=w388:refnum<queue>)
        n147 = disable-structure shown="启用" {
          disable-tunnel: [w396 w401] -> w383
          frame Disabled {
            n148 = Current VI's Path() -> (path=w399:path)
            n149 = Strip Path(path=w399) -> (stripped path=w398:path)  [unwired: 1 out]
            n150 = Build Path(base path=w398, name or relative path="HYLY003_main.vi" ("字符串")) -> (appended path=w396:path)
          }
          frame Enabled {
            n151 = vi-ref "UI_page111.vi"() -> (w400:refnum<vi>)
            n152 = property class="VI"(reference=w400) -> ("Name"=w401:string)  [unwired: 1 in, 2 out]
          }
        }
        n153 = Open VI Reference(type specifier VI Refnum (for type only)=refnum<vi> refnum ("类型说明符VI引用句柄（仅用于类型）"), vi path=w383, options=256, error in (no error)=w389) -> (vi reference=w384:refnum<vi>, error out=w382:errorcluster)  [unwired: 1 in, 1 out]
        n154 = call-by-ref "开始异步调用"(reference=w384, error in=w382, "传递队列输入"=w388, "notifier"=w390) -> (reference out=w378:refnum<vi>, error out=w381:errorcluster)  [unwired: 10 in]
        n155 = invoke on="XTab" class="XTab (strict)" method="AddPage.vi"(error in=w381, "PageViRefnum"=w378, "PageName"="控制页面" ("format string"), "Closeable (T)"=w376, "Detachable (T)"=w376) -> (error out=w391:errorcluster)  [unwired: 3 in, 7 out]
        n156 = Replace Array Subset(array=w380, new element=w378, index=0 ("索引")) -> (w379:refnum<vi>[])
        n157 = Bundle By Name(cluster=w392, "线程数组"=w379) -> (w393:T4)
        n158 = call <vilib>:"Add State(s) to Queue__jki_lib_state_machine.vi"("State(s) in (\"\")"=w395) -> ("States Out"=w394:string)  [unwired: 14 in]
      }
      frame "初始化:打开界面2" {
        w402 = FALSE ("Closeable (T)")
        # "Your code here.\n(You can make a copy of, or modify, this frame)"
        n159 = Unbundle By Name(w418) -> ("线程数组"=w406:refnum<vi>[], "notifier out"=w416:refnum<notifier>, "queue out"=w414:refnum<queue>)
        n160 = disable-structure shown="启用" {
          disable-tunnel: [w422 w427] -> w409
          frame Disabled {
            n161 = Current VI's Path() -> (path=w425:path)
            n162 = Strip Path(path=w425) -> (stripped path=w424:path)  [unwired: 1 out]
            n163 = Build Path(base path=w424, name or relative path="HYLY003_main.vi" ("字符串")) -> (appended path=w422:path)
          }
          frame Enabled {
            n164 = vi-ref "UI_page12.vi"() -> (w426:refnum<vi>)
            n165 = property class="VI"(reference=w426) -> ("Name"=w427:string)  [unwired: 1 in, 2 out]
          }
        }
        n166 = Open VI Reference(type specifier VI Refnum (for type only)=refnum<vi> refnum ("类型说明符VI引用句柄（仅用于类型）"), vi path=w409, options=256, error in (no error)=w415) -> (vi reference=w410:refnum<vi>, error out=w408:errorcluster)  [unwired: 1 in, 1 out]
        n167 = call-by-ref "开始异步调用"(reference=w410, error in=w408, "传递队列输入"=w414, "notifier"=w416) -> (reference out=w404:refnum<vi>, error out=w407:errorcluster)  [unwired: 10 in]
        n168 = invoke on="XTab" class="XTab (strict)" method="AddPage.vi"(error in=w407, "PageViRefnum"=w404, "PageName"="1553B主份" ("format string"), "Closeable (T)"=w402, "Detachable (T)"=w402) -> (error out=w417:errorcluster)  [unwired: 3 in, 7 out]
        n169 = Replace Array Subset(array=w406, new element=w404, index=0 ("索引")) -> (w405:refnum<vi>[])
        n170 = Bundle By Name(cluster=w418, "线程数组"=w405) -> (w419:T4)
        n171 = call <vilib>:"Add State(s) to Queue__jki_lib_state_machine.vi"("State(s) in (\"\")"=w421) -> ("States Out"=w420:string)  [unwired: 14 in]
      }
      frame "初始化:打开界面3" {
        w428 = FALSE ("Closeable (T)")
        # "Your code here.\n(You can make a copy of, or modify, this frame)"
        n172 = Unbundle By Name(w444) -> ("线程数组"=w432:refnum<vi>[], "notifier out"=w442:refnum<notifier>, "queue out"=w440:refnum<queue>)
        n173 = disable-structure shown="启用" {
          disable-tunnel: [w448 w453] -> w435
          frame Disabled {
            n174 = Current VI's Path() -> (path=w451:path)
            n175 = Strip Path(path=w451) -> (stripped path=w450:path)  [unwired: 1 out]
            n176 = Build Path(base path=w450, name or relative path="HYLY003_main.vi" ("字符串")) -> (appended path=w448:path)
          }
          frame Enabled {
            n177 = vi-ref "UI_page13.vi"() -> (w452:refnum<vi>)
            n178 = property class="VI"(reference=w452) -> ("Name"=w453:string)  [unwired: 1 in, 2 out]
          }
        }
        n179 = Open VI Reference(type specifier VI Refnum (for type only)=refnum<vi> refnum ("类型说明符VI引用句柄（仅用于类型）"), vi path=w435, options=256, error in (no error)=w441) -> (vi reference=w436:refnum<vi>, error out=w434:errorcluster)  [unwired: 1 in, 1 out]
        n180 = call-by-ref "开始异步调用"(reference=w436, error in=w434, "传递队列输入"=w440, "notifier"=w442) -> (reference out=w430:refnum<vi>, error out=w433:errorcluster)  [unwired: 10 in]
        n181 = invoke on="XTab" class="XTab (strict)" method="AddPage.vi"(error in=w433, "PageViRefnum"=w430, "PageName"="1553B备份" ("format string"), "Closeable (T)"=w428, "Detachable (T)"=w428) -> (error out=w443:errorcluster)  [unwired: 3 in, 7 out]
        n182 = Replace Array Subset(array=w432, new element=w430, index=0 ("索引")) -> (w431:refnum<vi>[])
        n183 = Bundle By Name(cluster=w444, "线程数组"=w431) -> (w445:T4)
        n184 = call <vilib>:"Add State(s) to Queue__jki_lib_state_machine.vi"("State(s) in (\"\")"=w447) -> ("States Out"=w446:string)  [unwired: 14 in]
      }
      frame "初始化:打开通讯线程" {
        n185 = vi-ref "CPCI_fifo.vi"() -> (w455:refnum<vi>)
        n186 = Unbundle By Name(w468) -> ("notifier out"=w459:refnum<notifier>, "queue out"=w454:refnum<queue>)
        n187 = flat-sequence {
          tunnel: w464 -> [w471]
          tunnel: [w471] -> w456
          frame #0 {
            n188 = Wait (ms)(milliseconds to wait=u32 100 ("等待时间（毫秒）")) -> ()  [unwired: 1 out]
          }
        }
        n189 = property class="VI"(reference=w455, error in=w456) -> (error out=w458:errorcluster, "Name"=w462:string)  [unwired: 1 out]
        n190 = Open VI Reference(type specifier VI Refnum (for type only)=refnum<vi> refnum ("类型说明符VI引用句柄（仅用于类型）"), vi path=w462, options=256, error in (no error)=w458) -> (vi reference=w460:refnum<vi>, error out=w457:errorcluster)  [unwired: 2 out]
        n191 = call-by-ref "开始异步调用"(reference=w460, error in=w457, "传递队列"=w454, "notifier"=w459) -> (reference out=w467:refnum<vi>, error out=w465:errorcluster)  [unwired: 10 in]
        n192 = Bundle By Name(cluster=w468, "通讯线程"=w467) -> (w466:T4)
        n193 = call <vilib>:"Add State(s) to Queue__jki_lib_state_machine.vi"("State(s) in (\"\")"=w470) -> ("States Out"=w469:string)  [unwired: 14 in]
      }
      frame "初始化:打开文件存储" {
        n194 = vi-ref "Save_file_txt_fifo.vi"() -> (w474:refnum<vi>)
        n195 = Unbundle By Name(w487) -> ("notifier out"=w478:refnum<notifier>, "queue out"=w473:refnum<queue>)
        n196 = flat-sequence {
          tunnel: w483 -> [w490]
          tunnel: [w490] -> w475
          frame #0 {
            n197 = Wait (ms)(milliseconds to wait=u32 100 ("等待时间（毫秒）")) -> ()  [unwired: 1 out]
          }
        }
        n198 = property class="VI"(reference=w474, error in=w475) -> (error out=w477:errorcluster, "Name"=w481:string)  [unwired: 1 out]
        n199 = Open VI Reference(type specifier VI Refnum (for type only)=refnum<vi> refnum ("类型说明符VI引用句柄（仅用于类型）"), vi path=w481, options=256, error in (no error)=w477) -> (vi reference=w479:refnum<vi>, error out=w476:errorcluster)  [unwired: 2 out]
        n200 = call-by-ref "开始异步调用"(reference=w479, error in=w476, "传递队列"=w473, "notifier"=w478) -> (reference out=w486:refnum<vi>, error out=w484:errorcluster)  [unwired: 10 in]
        n201 = Bundle By Name(cluster=w487, "txt引用"=w486) -> (w485:T4)
        n202 = call <vilib>:"Add State(s) to Queue__jki_lib_state_machine.vi"("State(s) in (\"\")"=w489) -> ("States Out"=w488:string)  [unwired: 14 in]
      }
      frame "---------- 反初始化----------" {
        n203 = call <vilib>:"Add State(s) to Queue__jki_lib_state_machine.vi"("State(s) in (\"\")"=w495) -> ("States Out"=w494:string)  [unwired: 14 in]
      }
      frame "反初始化：销毁数据寄存器" {
        n204 = call <vilib>:"Destroy.vi"("Register name"="VMC_Receive", "Error in"=w503) -> ("Error out"=w511:errorcluster)  [unwired: 12 in, 1 out]
        n205 = call <vilib>:"Destroy.vi"("Register name"="EFMC_Receive", "Error in"=w511) -> ("Error out"=w510:errorcluster)  [unwired: 12 in, 1 out]
        n206 = call <vilib>:"Destroy.vi"("Register name"="EFMC_Receive_Upload", "Error in"=w510) -> ("Error out"=w509:errorcluster)  [unwired: 12 in, 1 out]
        n207 = call <vilib>:"Destroy.vi"("Register name"="GNC_Receive_Upload", "Error in"=w509) -> ("Error out"=w508:errorcluster)  [unwired: 12 in, 1 out]
        n208 = call <vilib>:"Destroy.vi"("Register name"="GNC_Receive", "Error in"=w508) -> ("Error out"=w502:errorcluster)  [unwired: 12 in, 1 out]
        n209 = call <vilib>:"Destroy.vi"("Register name"="RT-Date-1", "Error in"=w502) -> ("Error out"=w501:errorcluster)  [unwired: 12 in, 1 out]
        n210 = call <vilib>:"Destroy.vi"("Register name"="RT-Date-2", "Error in"=w501) -> ("Error out"=w498:errorcluster)  [unwired: 12 in, 1 out]
        n211 = call <vilib>:"Destroy.vi"("Register name"="DC_Receive", "Error in"=w498) -> ("Error out"=w496:errorcluster)  [unwired: 12 in, 1 out]
        n212 = call <vilib>:"Destroy.vi"("Register name"="current_pack", "Error in"=w496) -> ("Error out"=w515:errorcluster)  [unwired: 12 in, 1 out]
        n213 = call <vilib>:"Destroy.vi"("Register name"="pack_num", "Error in"=w515) -> ("Error out"=w518:errorcluster)  [unwired: 12 in, 1 out]
        n214 = for {
          N: 48 -> [_]
          tunnel: "sensor" -> [w529]
          shift-right: [w525] -> w514
          shift-left: w518 -> [w526]
          i -> [w531]
          n215 = Number To Decimal String(number=w531, width (-)=i16 2 ("宽度(-)")) -> (decimal integer string=w528:string)
          n216 = Concatenate Strings(w529, w528) -> (w527:string)
          n217 = call <vilib>:"Destroy.vi"("Register name"=w527, "Error in"=w526) -> ("Error out"=w525:errorcluster)  [unwired: 12 in, 1 out]
        }
        n218 = call <vilib>:"Add State(s) to Queue__jki_lib_state_machine.vi"("State(s) in (\"\")"=w524, "State(s) at Back (\"\")"="Macro: Exit") -> ("States Out"=w523:string)  [unwired: 13 in]
        n219 = call <vilib>:"DestroyAll.vi"("Error in"=w514) -> ("Error out"=w513:errorcluster)  [unwired: 13 in, 1 out]
      }
    }
  }
